vi "Chamber controller Dec 1 2016 no K2420.vi"() -> ()   [LabVIEW 2014]
uses:
  <vilib>/Instr/_visa.llb/VISA Configure Serial Port (Instr).vi
  Environmental Chamber LabVIEW and Instruments/Drivers and Software/Keithley 2100 Series/Public/Configure/Configure 2 Wire Resistance.vi
  <vilib>/Utility/file.llb/Write To Spreadsheet File (string).vi
  <vilib>/Utility/file.llb/Read From Spreadsheet File (string).vi
  Environmental Chamber LabVIEW and Instruments/Drivers and Software/keithley_6430/Keithley 6430/Public/Data/Read (Single Point).vi
  Environmental Chamber LabVIEW and Instruments/Drivers and Software/keithley_6430/Keithley 6430/Keithley 6430.lvlib
  Environmental Chamber LabVIEW and Instruments/Drivers and Software/Keithley 2100 Series/Keithley 2100 Series.lvlib
panel:
  in  "Arduino COMs":T1={"Arduino 1"="COM23", "Arduino 2"="COM24", "Arduino 3"="COM25", "Arduino 4"="COM26", "Arduino 5"="COM27", "Arduino 6"="COM28"}
  out "saving data?":bool
  out "ArduinoQCM\ncluster":T2 caption="Arduino QCM" {"6" format="%_8g"; "5" format="%_8g"; "4" format="%_8g"; "3" format="%_8g"; "2" format="%_8g"; "1" format="%#_10g"}
  in  "Data logging settings":T3={"Save during sequence only"=TRUE, "Save now"=FALSE, "sec between data points"=0.0, "Current data file path"=path "", "Save sample names"={"QCM1"="", "QCM2"="", "QCM3"="", "QCM4"="", "QCM5"="", "QCM6"="", "SRS"="", "K-2420"="", "K-6430"="", "K-2100"=""}, "Experiment Notes"=""} {"sec between data points" min=0.0 max=30.0 format="%#_13g"}
  in  "Sequence cluster":T4={"Save sequence"=FALSE, "Clear sequence"=FALSE, "Import sequence file"=FALSE, "Tare elapsed time"=TRUE, "Run Sequence"=FALSE, "Stop program when sequence ends"=TRUE, "User-defined\nsequence"=[], "Sequence end time"="", "Sequence\npreview"=[], "Current\nstep"=0, "Jump to next step"=FALSE} caption="Sequence settings"
  in  "Pressure parameters cluster":T5={"valve % open"=100.0, "Desired pressure"=0.0, "Vapor sccm"=0.0, "Gas sccm"=0.0, "Valve mode"=enum."% Open", "Pressure Mode"=enum."Abs. pressure", "analyte partial pressure"=23.8, "Turbo pump\nauto on"=TRUE, "Valve position (%)"=0.0, "read pressure"=0.0, "read vapor flow"=0.0, "read gas flow"=0.0, "pressure chart"={"pressure"=0.0}} caption="Pressure settings" {"read gas flow" format="%#_3g"; "read vapor flow" format="%#_3g"; "read pressure" format="%#_7f"; "Valve position (%)" format="%#_3g"; "analyte partial pressure" min=0.0 max=100.0 step=5.0; "Gas sccm" min=0 max=200 step=5; "Vapor sccm" min=0 max=200 step=5; "Desired pressure" min=0.0 max=760.0 step=5.0; "valve % open" min=0.0 max=100.0 step=5.0 format="%#_2f"}
  out "J-KEM temp chart":dbl(graph)
  out "Elapsed time (min)":dbl
  out "State date/time":string caption="Start time"
  out "K-2100 (Ohm)":cluster{"Measurement":dbl}(graph) caption="K-2100"
  out "K-6430":cluster{"Measurement":dbl}(graph)
  out "K-2420":cluster{"Resistance":sgl}(graph)
  in  "Gate time (sec)":enum16{"0.1", "1.0 ", "10"}(ring)=enum."1.0 "
  out "Hz":dbl format="%.7f"
  out "QCM plot":T6(graph)
  in  "Stop":bool
  in  "Clear all charts":bool
  out "O2 sensor output":dbl[](array[numeric]) caption="atm\nTorr"
  in  "rapidox O2 Sensor":bool
  in  "setnag O2 Pump":bool
  in  "Baud Rate 2":i32(ring)=2 items=["2400", "4800", "9600", "19200", "38400", "57600", "115200"]
  in  "Com Port":i32(ring) items=["Com 1", "Com 2", "Com 3", "Com 4", "Com 5", "Com 6", "COM 7", "COM 8", "COM 9", "COM 10", "COM 11", "COM 12", "com 13", "COM 14"]
  in  "Com Port 2":i32(ring) items=["Com 1", "Com 2", "Com 3", "Com 4", "Com 5", "Com 6", "COM 7", "COM 8", "COM 9", "COM 10", "COM 11", "COM 12", "com 13", "COM 14"]
  out "Waveform Chart":cluster{dbl}(graph)
  out "O2 Concentration (PPM)":dbl
  out "Waveform Chart 6":cluster{dbl}(graph)
  # "Currently Unused"
  # "100%"
  # "SRS"
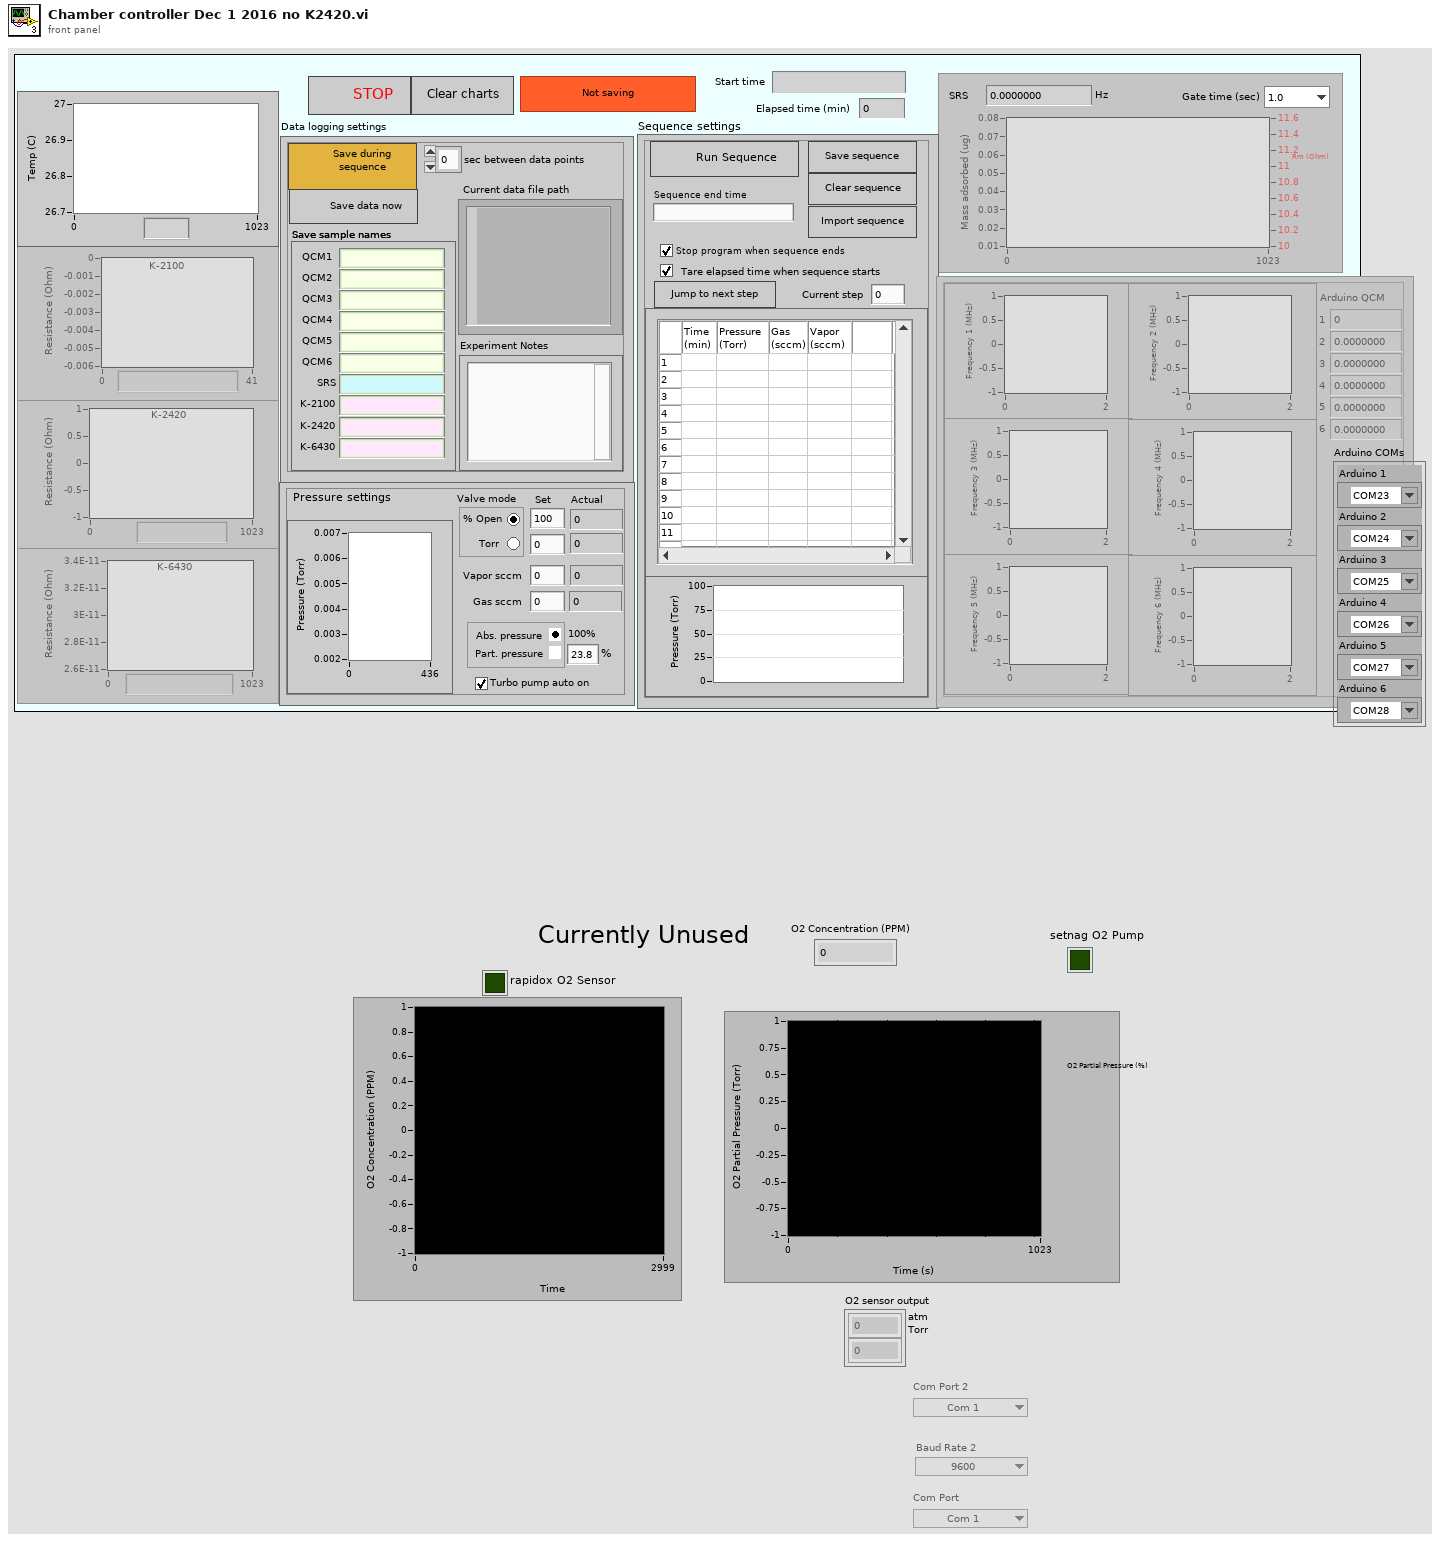
[diagram p1: front panel]
types:
  T1 = cluster{"Arduino 1":refnum<visa-resource-name>, "Arduino 2":refnum<visa-resource-name>, "Arduino 3":refnum<visa-resource-name>, "Arduino 4":refnum<visa-resource-name>, "Arduino 5":refnum<visa-resource-name>, "Arduino 6":refnum<visa-resource-name>}
  T2 = cluster{"arduino qcm 1":dbl, "1":dbl, "arduino qcm 2":dbl, "2":dbl, "arduino qcm 3":dbl, "3":dbl, "arduino qcm 4":dbl, "4":dbl, "arduino qcm 5":dbl, "5":dbl, "arduino qcm 6":dbl, "6":dbl}
  T3 = cluster{"Save during sequence only":bool, "Save now":bool, "sec between data points":dbl, "Current data file path":path, "Save sample names":cluster{"QCM1":string, "QCM2":string, "QCM3":string, "QCM4":string, "QCM5":string, "QCM6":string, "SRS":string, "K-2420":string, "K-6430":string, "K-2100":string}, "Experiment Notes":string}
  T4 = cluster{"Save sequence":bool, "Clear sequence":bool, "Import sequence file":bool, "Tare elapsed time":bool, "Run Sequence":bool, "Stop program when sequence ends":bool, "User-defined\nsequence":string[][], "Sequence end time":string, "Sequence\npreview":cluster{dbl[], dbl[]}[], "Current\nstep":i32, "Jump to next step":bool}
  T5 = cluster{"valve % open":dbl, "Desired pressure":dbl, "Vapor sccm":sgl, "Gas sccm":sgl, "Valve mode":enum32{"% Open", "Torr "}, "Pressure Mode":enum32{"Abs. pressure", " Part. pressure"}, "analyte partial pressure":dbl, "Turbo pump\nauto on":bool, "Valve position (%)":dbl, "read pressure":dbl, "read vapor flow":dbl, "read gas flow":dbl, "pressure chart":cluster{"pressure":dbl}}
  T6 = cluster{"Numeric Control":dbl, "Resistance out":dbl}
  T7 = cluster{"Keithley 6430":bool, "J-KEM":bool, "Keithley 2420":bool, "Keithley 2100":bool, "SRS QCM":bool, "Pressure control":bool, "Arduino":bool}
  T8 = enum8{"Enabled", "Disabled", "Disabled and Grayed Out"}
  T9 = enum16{"open", "open or create", "create or replace", "create", "open (read only)"}
  T10 = enum16{"no parity", "odd parity", "even parity", "mark parity", "space parity"}
  T11 = cluster{"String":string, "String":string, "String":string}
  T12 = cluster{"task out":refnum<k21>, "error out":errorcluster, "task out":refnum<k21>, "error out":errorcluster, "task out":refnum<k21>, "error out":errorcluster, "VISA resource name":refnum<visa-resource-name>, "error out":errorcluster}
  T13 = cluster{"task out":refnum<k21>, "error out":errorcluster, "task out":refnum<k21>, "error out":errorcluster, "task out":refnum<k21>, "error out":errorcluster, "VISA resource name out":refnum<visa-resource-name>, "error out":errorcluster}
  T14 = cluster{bool, "VISA resource name":refnum<visa-resource-name>, "error out":errorcluster}
  T15 = cluster{bool, "VISA resource name out":refnum<visa-resource-name>, "error out":errorcluster}
  T16 = cluster{"VISA resource name out":refnum<visa-resource-name>, "error out":errorcluster, "VISA resource name out":refnum<visa-resource-name>, "error out":errorcluster, "VISA resource name out":refnum<visa-resource-name>, "error out":errorcluster, "VISA resource name out":refnum<visa-resource-name>, "error out":errorcluster, "VISA resource name out":refnum<visa-resource-name>, "error out":errorcluster, "VISA resource name out 2":refnum<visa-resource-name>, "error out 2":errorcluster}
  T17 = cluster{bool, cluster{"task out":refnum<k21>, "error out":errorcluster, "task out":refnum<k21>, "error out":errorcluster, "task out":refnum<k21>, "error out":errorcluster, "VISA resource name out":refnum<visa-resource-name>, "error out":errorcluster}}
  T18 = cluster{"f":dbl, "f":dbl, "f":dbl, "f":dbl, "f":dbl, "f 2":dbl}
  T19 = cluster{"Boolean":bool, "VISA resource name out":refnum<visa-resource-name>, "error out":errorcluster}
  T20 = cluster{bool, "VISA out":refnum<visa-resource-name>, "error out":errorcluster}
  T21 = cluster{"Boolean":bool, "VISA out":refnum<visa-resource-name>, "error out":errorcluster}
  T22 = cluster{"Numeric Control":dbl, "Cluster":cluster{"Numeric Control":dbl}, "String":string, "error out":errorcluster}
  T23 = cluster{bool, "Com Port":i32, "Numeric Control out":dbl}
  T24 = cluster{"Arduino address":refnum<visa-resource-name>, "error in (no error)":errorcluster, "Arduino address 2":refnum<visa-resource-name>, "error in (no error) 2":errorcluster, "Arduino address 3":refnum<visa-resource-name>, "error in (no error) 3":errorcluster, "Arduino address 4":refnum<visa-resource-name>, "error in (no error) 4":errorcluster, "Arduino address 5":refnum<visa-resource-name>, "error in (no error) 5":errorcluster, "Arduino address 6":refnum<visa-resource-name>, "error in (no error) 6":errorcluster}
  T25 = cluster{"mean":string, "mean":string, "mean":string, "mean":string, "mean":string, "mean":string}
  T26 = cluster{"String data out":string, string, string, string}
  T27 = cluster{"valve % open":dbl, "Desired pressure":dbl, "Vapor sccm":sgl, "Gas sccm":sgl, "Valve mode":enum32{"% Open", "Torr "}, "Pressure Mode":enum32{"Abs. pressure", " Part. pressure"}, "analyte partial pressure":dbl, "Turbo pump\nauto on":bool}
  T28 = cluster{"User-defined\nsequence":string[][], "Present (s)":dbl, "current  step # in":i32, "sequence end time in":timestamp}
  T29 = cluster{"current  step # in":i32, "sequence end time in":timestamp, "Boolean":bool}
  T30 = cluster{"press/RH/gas/vapor":cluster{"pressure":string, "RH":string, "gas flow":string, "vapor flow":string}, "Cluster":cluster{"Valve position (%)":dbl, "read pressure":dbl, "read vapor flow":dbl, "read gas flow":dbl}}
  T31 = cluster{"Boolean":bool, "DAQ IDs in":cluster{"task out":refnum<k21>, "error out":errorcluster, "task out":refnum<k21>, "error out":errorcluster, "task out":refnum<k21>, "error out":errorcluster, "VISA Refnum out":refnum<visa-resource-name>, "error out":errorcluster}}
  T32 = cluster{"mean":dbl, "mean":dbl, "mean":dbl, "mean":dbl, "mean":dbl, "mean":dbl}
  T33 = cluster{"f":dbl, "f":dbl, "f":dbl, "f":dbl, "f":dbl}[]
  T34 = cluster{"pressure":string, "RH":string, "gas flow":string, "vapor flow":string}
  T35 = cluster{"Valve position (%)":dbl, "read pressure":dbl, "read vapor flow":dbl, "read gas flow":dbl}
  T36 = cluster{"mean":dbl, "mean":dbl, "mean":dbl, "mean":dbl, "mean":dbl, "mean":dbl, "mean":dbl, "mean":dbl, "mean":dbl, "mean":dbl, "mean":dbl, "mean":dbl}
  T37 = cluster{"QCM1":string, "QCM2":string, "QCM3":string, "QCM4":string, "QCM5":string, "QCM6":string, "SRS":string, "K-2420":string, "K-6430":string, "K-2100":string}
  T38 = cluster{"task out":refnum<k21>, "error out":errorcluster, "task out":refnum<k21>, "error out":errorcluster, "task out":refnum<k21>, "error out":errorcluster, "VISA Refnum out":refnum<visa-resource-name>, "error out":errorcluster}
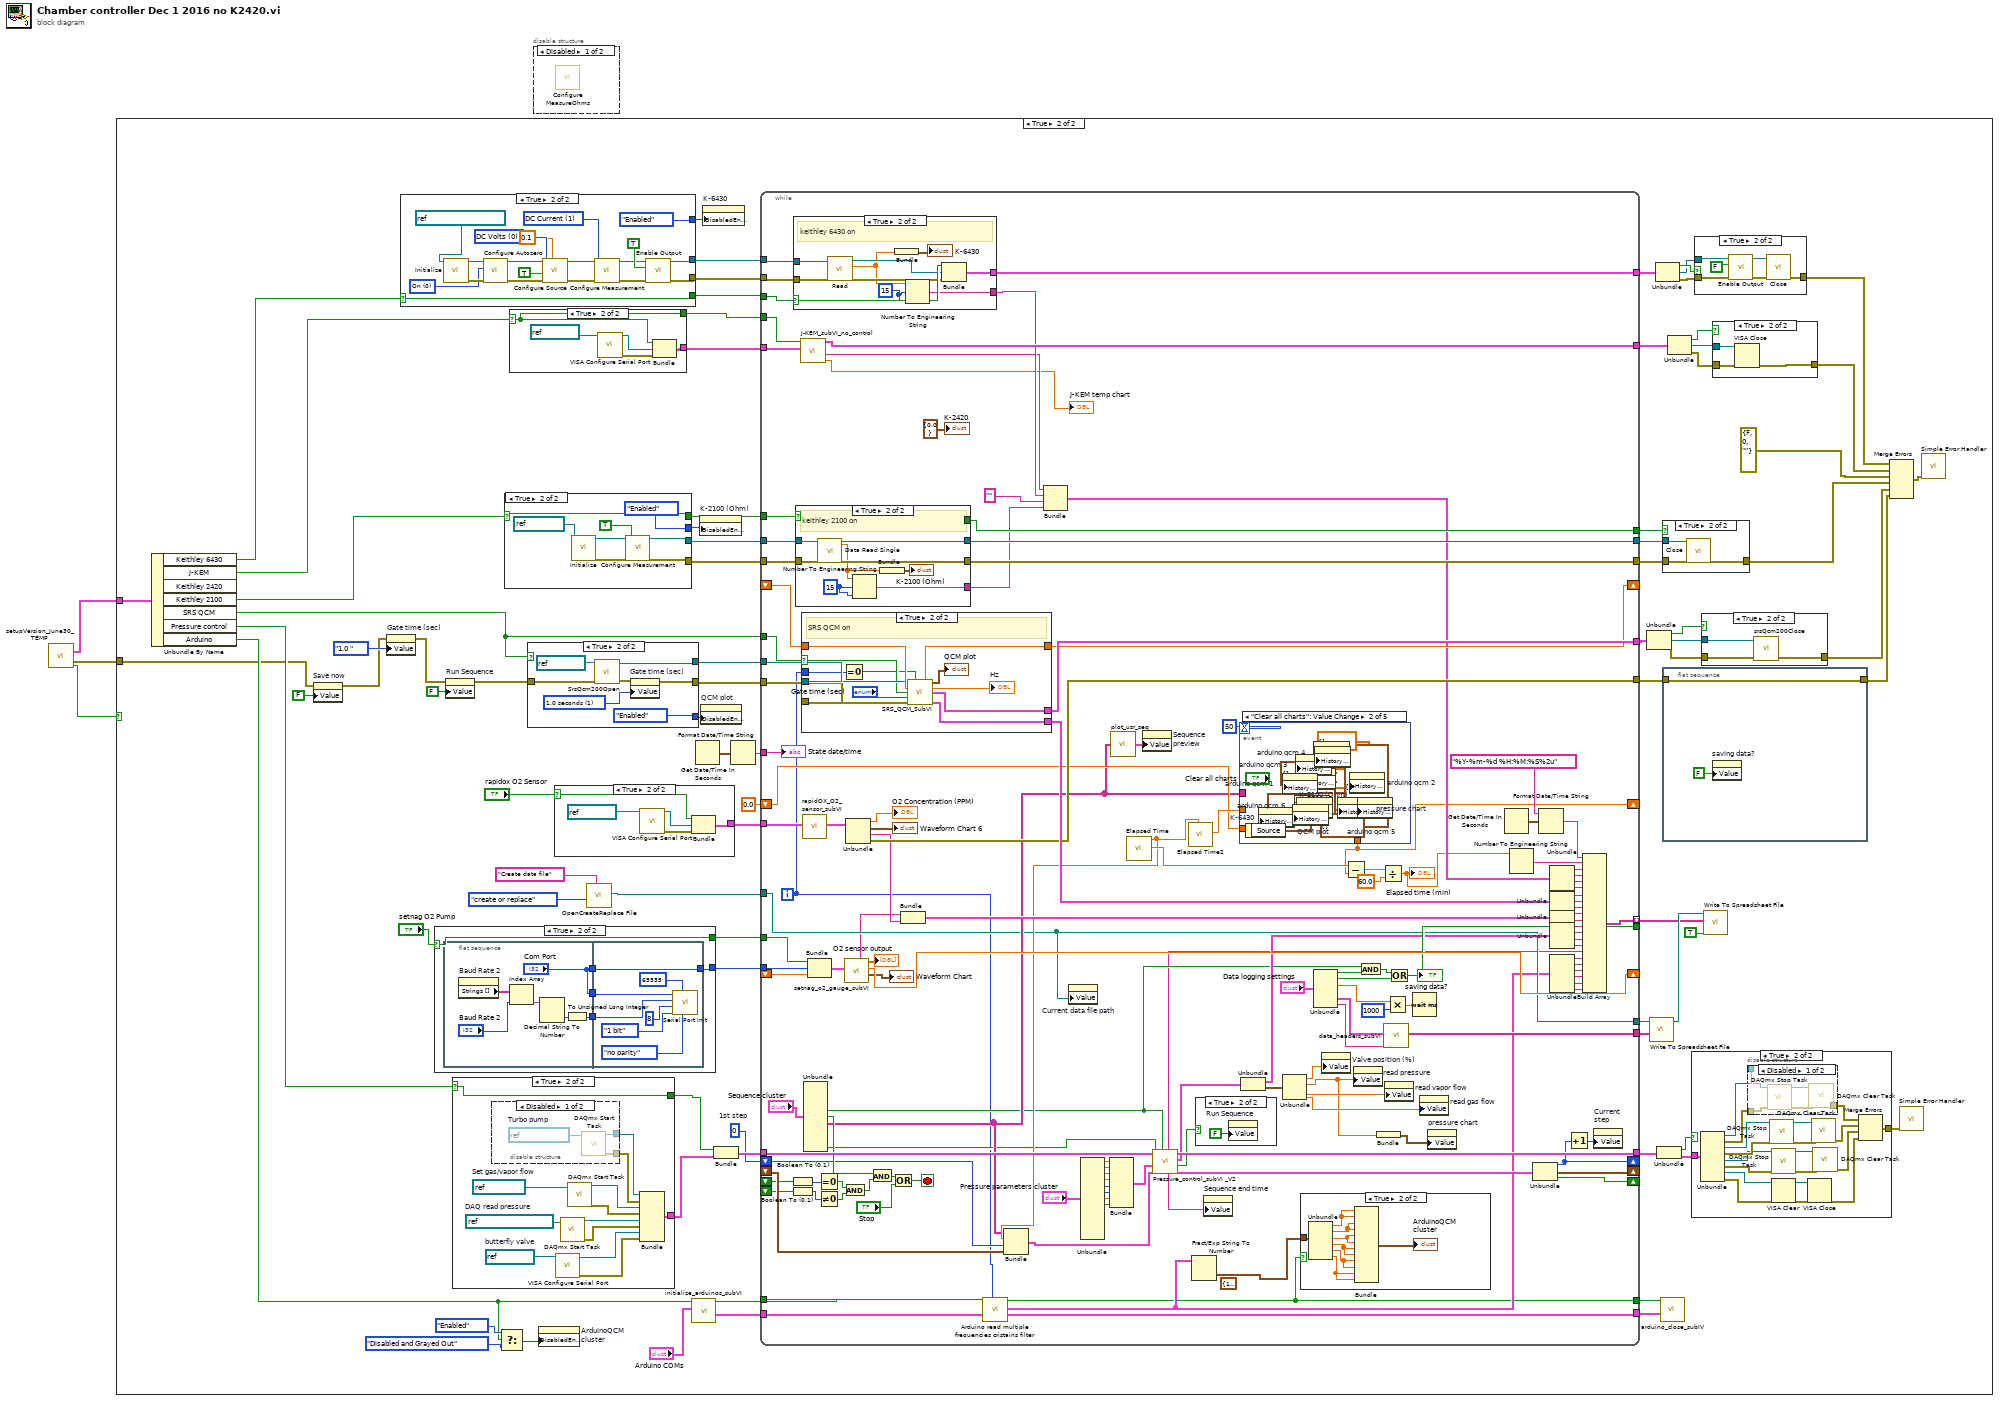
[diagram p0: block diagram]
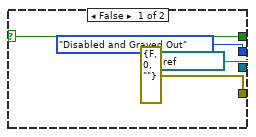
[diagram p5: hidden frame]
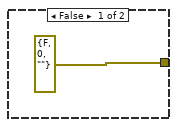
[diagram p6: hidden frame]
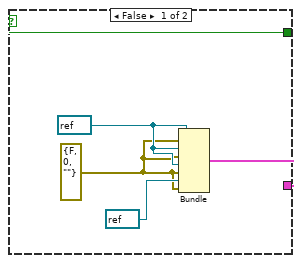
[diagram p8: hidden frame]
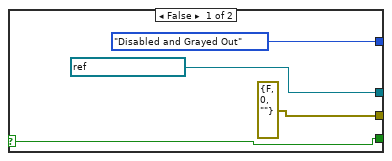
[diagram p11: hidden frame]
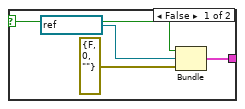
[diagram p12: hidden frame]
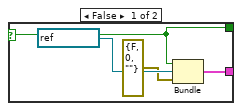
[diagram p14: hidden frame]
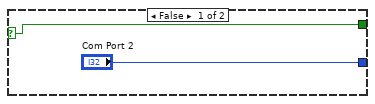
[diagram p15: hidden frame]
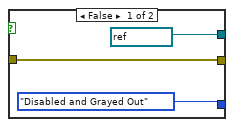
[diagram p17: hidden frame]
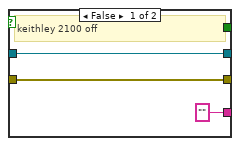
[diagram p20: hidden frame]
diagram:
  n1 = call "setupVersion_June30_TEMP.vi"() -> ("Instruments on/off"=w1:T7, "error IO"=w2:errorcluster, "OK"=w3:bool)  [unwired: 13 in]
  n2 = case shown="True" w3 {
    tunnel: w2 -> [_ w9]
    tunnel: w1 -> [_ w16]
    frame False {
    }
    frame True {
      w28 = 0  # 1st step
      n3 = Unbundle By Name(w16) -> ("Keithley 6430"=w15:bool, "J-KEM"=w14:bool, "Keithley 2100"=w13:bool, "SRS QCM"=w12:bool, "Pressure control"=w11:bool, "Arduino"=w10:bool)  [unwired: 1 out]
      n4 = property on="Save now" class="Bool (strict)"(error in=w9, "Value"=FALSE) -> (error out=w8:errorcluster)  [unwired: 1 in, 1 out]
      n5 = property on="Gate time (sec)" class="Enum (strict)"(error in=w8, "Value"=enum16{"0.1", "1.0 ", "10"}."1.0 " ("Gate time (sec)")) -> (error out=w17:errorcluster)  [unwired: 1 in, 1 out]
      n6 = case shown="True" w15 {
        selector: w15 -> [w158 w168]
        tunnel: [refnum<visa-resource-name> "GPIB0::29::INSTR" ("VISA resource name") w177] -> w59
        tunnel: [errorcluster {"status"=FALSE, "code"=0, "source"=""} ("error out") w178] -> w58
        tunnel: [T8."Disabled and Grayed Out" ("Disabled") T8."Enabled" ("Disabled")] -> w53
        tunnel: [w158 w168] -> w47
        frame False {
        }
        frame True {
          w163 = u16 1 items=["DC Volts", "DC Current"] ("Measure Function (1: DC Current)")
          w169 = u16 0 items=["DC Volts", "DC Current"] ("Source Function (0: DC Volts)")
          w174 = u16 0 items=["On", "Off", "Once"] ("Autozero  (0: On)")
          n7 = call "Initialize.vi"("VISA resource name"=refnum<visa-resource-name> "GPIB0::29::INSTR") -> ("error out"=w175:errorcluster, "VISA resource name out"=w176:refnum<visa-resource-name>)  [unwired: 4 in, 5 out]
          n8 = call "Configure Autozero.vi"("error in (no error)"=w175, "Autozero  (0: On)"=w174, "VISA resource name"=w176) -> ("error out"=w171:errorcluster, "VISA resource name out"=w172:refnum<visa-resource-name>)  [unwired: 7 in]
          n9 = call "Configure Source.vi"("V-Source Level [V]"=0.1, "error in (no error)"=w171, "Auto Range (T:Enable)"=TRUE, "Source Function (0: DC Volts)"=w169, "VISA resource name"=w172) -> ("error out"=w165:errorcluster, "VISA resource name out"=w167:refnum<visa-resource-name>)  [unwired: 5 in]
          n10 = call "Configure Measurement.vi"("error in (no error)"=w165, "Measure Function (1: DC Current)"=w163, "VISA resource name"=w167) -> ("error out"=w164:errorcluster, "VISA resource name out"=w166:refnum<visa-resource-name>)  [unwired: 7 in]
          n11 = call "Enable Output.vi"("error in (no error)"=w164, "Enable Output (F:Off)"=TRUE ("Output (F:Off)"), "VISA resource name"=w166) -> ("error out"=w178:errorcluster, "VISA resource name out"=w177:refnum<visa-resource-name>)  [unwired: 7 out]
        }
      }
      n12 = case shown="True" "setnag O2 Pump" {
        selector: "setnag O2 Pump" -> [w203 w205]
        tunnel: ["Com Port 2" w206] -> w81
        tunnel: [w203 w205] -> w36
        frame False {
        }
        frame True {
          n13 = flat-sequence {
            tunnel: ["Com Port"] -> w209
            tunnel: [w211] -> w208
            tunnel: ["Com Port"] -> w207
            tunnel: w209 -> [w217]
            tunnel: w208 -> [w216]
            tunnel: w207 -> [w218]
            tunnel: [w218] -> w206
            frame #0 {
              n14 = property on="Baud Rate 2" class="Ring (strict)"() -> ("Strings []"=w213:string[])  [unwired: 2 in, 2 out]
              n15 = Index Array(array=w213, index="Baud Rate 2") -> (element=w214:string)
              n16 = Decimal String To Number(string=w214) -> (number=w212:i32)  [unwired: 2 in, 1 out]
              n17 = To Unsigned Long Integer(number=w212) -> (unsigned 32bit integer=w211:u32)
            }
            frame #1 {
              n18 = call <vilib>:"Serial Port Init.vi"("parity"=T10."no parity", "buffer size"=u16 65535, "stop bits"=enum16{"1 bit", "1.5 bits", "2 bits"}."1 bit", "data bits"=u16 8, "baud rate"=w216, "port number"=w217) -> ()  [unwired: 1 in, 1 out]
            }
          }
        }
      }
      n19 = property on="Run Sequence" class="Bool (strict)"(error in=w17, "Value"=FALSE) -> (error out=w23:errorcluster)  [unwired: 1 in, 1 out]
      n20 = case shown="True" w11 {
        selector: w11 -> [w130 w135]
        tunnel: [w131 w137] -> w30
        tunnel: [w130 w135] -> w31
        frame False {
          w133 = refnum<k21> refnum ("task out")
          w132 = errorcluster {"status"=FALSE, "code"=0, "source"=""} ("error out")
          n21 = Bundle("task out"=w133, "error out"=w132, "task out"=w133, "error out"=w132, "task out"=w133, "error out"=w132, "VISA resource name"=refnum<visa-resource-name> refnum, "error out"=w132) -> (w131:T12)  [unwired: 1 in]
        }
        frame True {
          w145 = refnum<visa-resource-name> "COM5"  # butterfly valve
          w146 = refnum<k21> "Setflow"  # Set gas/vapor flow
          w147 = refnum<k21> "AllDaqReadings"  # DAQ read pressure
          n22 = disable-structure shown="Disabled" {
            disable-tunnel: [w149 _] -> w144
            disable-tunnel: [w148 _] -> w143
            frame Disabled {
              w150 = refnum<k21> "TurboON"  # Turbo pump
              n23 = call <vilib>:"DAQmx Start Task.vi"("task/channels in"=w150) -> ("task out"=w149:refnum<k21>, "error out"=w148:errorcluster)  [unwired: 13 in]
            }
            frame Enabled {
            }
          }
          n24 = call-poly "VISA Configure Serial Port"("VISA resource name"=w145) -> ("VISA resource name out"=w138:refnum<visa-resource-name>, "error out"=w136:errorcluster)  [unwired: 13 in]
          n25 = call <vilib>:"DAQmx Start Task.vi"("task/channels in"=w147) -> ("task out"=w140:refnum<k21>, "error out"=w139:errorcluster)  [unwired: 13 in]
          n26 = call <vilib>:"DAQmx Start Task.vi"("task/channels in"=w146) -> ("task out"=w142:refnum<k21>, "error out"=w141:errorcluster)  [unwired: 13 in]
          n27 = Bundle("task out"=w144, "error out"=w143, "task out"=w142, "error out"=w141, "task out"=w140, "error out"=w139, "VISA resource name out"=w138, "error out"=w136) -> (w137:T13)  [unwired: 1 in]
        }
      }
      n28 = Select(t=T8."Enabled" ("Disabled"), s=w10, f=T8."Disabled and Grayed Out" ("Disabled")) -> (s? t:f=w22:T8)
      n29 = case shown="True" w13 {
        selector: w13 -> [w93 w98]
        tunnel: [refnum<visa-resource-name> "K-2100" ("VISA resource name out") w101] -> w45
        tunnel: [errorcluster {"status"=FALSE, "code"=0, "source"=""} ("error out") w100] -> w44
        tunnel: [w93 w98] -> w43
        tunnel: [T8."Disabled and Grayed Out" ("Disabled") T8."Enabled" ("Disabled")] -> w38
        frame False {
        }
        frame True {
          n30 = call "Initialize.vi"("VISA resource name"=refnum<visa-resource-name> "K-2100") -> ("VISA resource name out"=w102:refnum<visa-resource-name>, "error out"=w99:errorcluster)  [unwired: 17 in]
          n31 = call-poly "Configure Measurement.vi"("VISA resource name"=w102, "error in (no error)"=w99, "Auto Range? (T: Auto)"=TRUE) -> ("VISA resource name out"=w101:refnum<visa-resource-name>, "error out"=w100:errorcluster)  [unwired: 15 in]
        }
      }
      n32 = case shown="True" w14 {
        selector: w14 -> [w194 w199]
        tunnel: [w195 w200] -> w75
        tunnel: [w194 w199] -> w69
        frame False {
          n33 = Bundle(w194, "VISA resource name"=refnum<visa-resource-name> "COM3", "error out"=errorcluster {"status"=FALSE, "code"=0, "source"=""}) -> (w195:T14)  [unwired: 1 in]
        }
        frame True {
          n34 = call-poly "VISA Configure Serial Port"("VISA resource name"=refnum<visa-resource-name> "COM3") -> ("VISA resource name out"=w201:refnum<visa-resource-name>, "error out"=w198:errorcluster)  [unwired: 13 in]
          n35 = Bundle(w199, "VISA resource name out"=w201, "error out"=w198) -> (w200:T15)  [unwired: 1 in]
        }
      }
      n36 = case shown="True" w12 {
        tunnel: [refnum<visa-resource-name> "COM6" ("VISA in") w233] -> w83
        tunnel: [w228 w230] -> w82
        tunnel: w23 -> [w228 w235]
        tunnel: [T8."Disabled and Grayed Out" ("Disabled") T8."Enabled" ("Disabled")] -> w54
        frame False {
        }
        frame True {
          w232 = u16 1 items=["0.1 seconds", "1.0 seconds", "10.0 seconds"] ("Gate time")
          n37 = call "SrsQcm200Open.vi"("error in"=w235, "VISA in"=refnum<visa-resource-name> "COM6") -> ("error out"=w231:errorcluster, "VISA out"=w233:refnum<visa-resource-name>)  [unwired: 3 in]
          n38 = property on="Gate time (sec)" class="Enum (strict)"(error in=w231, "Value"=w232) -> (error out=w230:errorcluster)  [unwired: 1 in, 1 out]
        }
      }
      n39 = property on="ArduinoQCM\ncluster" class="Clust (strict)"("DisabledEnum"=w22) -> ()  [unwired: 2 in, 2 out]
      n40 = case shown="True" "rapidox O2 Sensor" {
        selector: "rapidox O2 Sensor" -> [w181 w186]
        tunnel: [w182 w187] -> w65
        frame False {
          n41 = Bundle(w181, "VISA resource name"=refnum<visa-resource-name> "COM7", "error out"=errorcluster {"status"=FALSE, "code"=0, "source"=""}) -> (w182:T14)  [unwired: 1 in]
        }
        frame True {
          n42 = call-poly "VISA Configure Serial Port"("VISA resource name"=refnum<visa-resource-name> "COM7") -> ("VISA resource name out"=w188:refnum<visa-resource-name>, "error out"=w185:errorcluster)  [unwired: 13 in]
          n43 = Bundle(w186, "VISA resource name out"=w188, "error out"=w185) -> (w187:T15)  [unwired: 1 in]
        }
      }
      n44 = call "OpenCreateReplace File.vi"("prompt"="Create data file", "function (open:0)"=T9."create or replace") -> ("new file path"=w46:path)  [unwired: 6 in, 3 out]
      n45 = call "initialize_arduinos_subVI.vi"("arduino 1-6 addresses"="Arduino COMs", "arduinos on?"=w10) -> ("arduino addresses/errors"=w32:T16, "arduinos on/off"=w51:bool)  [unwired: 8 in]
      n46 = Get Date/Time In Seconds() -> (seconds since 1Jan1904=w85:timestamp)
      n47 = property on="K-2100 (Ohm)" class="WFChart (strict)"("DisabledEnum"=w38) -> ()  [unwired: 2 in, 2 out]
      n48 = property on="QCM plot" class="WFChart (strict)"("DisabledEnum"=w54) -> ()  [unwired: 2 in, 2 out]
      n49 = property on="K-6430" class="WFChart (strict)"("DisabledEnum"=w53) -> ()  [unwired: 2 in, 2 out]
      n50 = Bundle(w31, w30) -> (w29:T17)  [unwired: 1 in]
      n51 = Format Date/Time String(seconds (now)=w85) -> (date/time string=w35:string)  [unwired: 2 in]
      n52 = while {
        shift-right: [w377] -> _
        shift-left: _ -> [w313]
        tunnel: [w365] -> w52 mode=indexing if=w334
        tunnel: w83 -> [w376]
        tunnel: w82 -> [w375]
        tunnel: w12 -> [w374]
        tunnel: w36 -> [w315]
        tunnel: w81 -> [w316]
        tunnel: [w373] -> w79
        tunnel: w75 -> [w372]
        tunnel: [w371] -> w74
        tunnel: w69 -> [w370]
        tunnel: w65 -> [w323]
        tunnel: [w319] -> w6
        tunnel: [w255] -> w64
        tunnel: w46 -> [w255]
        shift-right: [w363] -> _
        shift-left: _ -> [w364]
        tunnel: w59 -> [w369]
        tunnel: w58 -> [w368]
        tunnel: [w367] -> w57
        tunnel: [w334] -> _
        tunnel: w51 -> [w242]
        tunnel: w32 -> [w245]
        tunnel: [w241] -> w49
        tunnel: [w243] -> w50
        tunnel: [w351] -> w48
        tunnel: w47 -> [w346]
        tunnel: w45 -> [w333]
        tunnel: w44 -> [w332]
        tunnel: w43 -> [w331]
        tunnel: [w330] -> w42
        tunnel: [w329] -> w41
        tunnel: [w328] -> w40
        shift-right: [w307] -> _
        shift-left: 0.0 ("Elapsed Time (s)") -> [w308]
        tunnel: w35 -> [w298]
        tunnel: w29 -> [w280]
        shift-right: [w250] -> _
        shift-left: w28 -> [w269]
        shift-right: [w275] -> _
        shift-left: _ -> [w273]
        shift-right: [w274] -> _
        shift-left: _ -> [w272]
        shift-left: _ -> [w271]
        tunnel: [w267] -> w27
        i -> [w240]
        stop <- w336 stop-if-true
        (unwired) T18 {"f"=1000000.0, "f"=1000000.0, "f"=1000000.0, "f"=1000000.0, "f"=1000000.0, "f 2"=1000000.0} ("y")
        n53 = Boolean To (0,1)(Boolean=w272) -> (0, 1=w344:i16)
        n54 = Boolean To (0,1)(Boolean=w271) -> (0, 1=w343:i16)
        n55 = case "Keithley 6430" shown="True" w346 {
          selector: w346 -> [w412 w423]
          tunnel: w369 -> [w411 w420]
          tunnel: w368 -> [w410 w419]
          tunnel: ["" w422] -> w318
          tunnel: [w409 w421] -> w367
          frame False {
            # "keithley 6430 off"
            n56 = Bundle(w412, "VISA resource name out"=w411, "error out"=w410) -> (w409:T15)  [unwired: 1 in]
          }
          frame True {
            w414 = i16 15 ("width (-)")
            # "keithley 6430 on"
            n57 = call-poly "Read.vi"("error in (no error)"=w419, "VISA resource name"=w420) -> ("error out"=w418:errorcluster, "Measurement"=w416:dbl, "VISA resource name out"=w417:refnum<visa-resource-name>)  [unwired: 1 in, 6 out]
            n58 = Bundle("Measurement"=w416) -> (→"K-6430":cluster{"Measurement":dbl})  [unwired: 1 in]
            n59 = Number To Engineering String(2:w414, 3:w414, 4:w416) -> (0:w422:string)  [unwired: 1 in]
            n60 = Bundle(w423, "VISA resource name out"=w417, "error out"=w418) -> (w421:T15)  [unwired: 1 in]
          }
        }
        n61 = case shown="True" w331 {
          selector: w331 -> [w388 w393]
          tunnel: [w389 w400] -> w329
          tunnel: [w390 w399] -> w328
          tunnel: w333 -> [w389 w398]
          tunnel: w332 -> [w390 w397]
          tunnel: ["" w395] -> w317
          tunnel: [w388 w393] -> w330
          frame False {
            # "keithley 2100 off"
          }
          frame True {
            w392 = i16 15 ("width (-)")
            # "keithley 2100 on"
            n62 = call "Data Read Single.vi"("VISA resource name"=w398, "error in (no error)"=w397) -> ("VISA resource name out"=w400:refnum<visa-resource-name>, "Measurement"=w396:dbl, "error out"=w399:errorcluster)  [unwired: 15 in]
            n63 = Number To Engineering String ("elapsed time (min)")(2:w392, 3:w392, 4:w396) -> (0:w395:string)  [unwired: 1 in]
            n64 = Bundle("Measurement"=w396) -> (→"K-2100 (Ohm)":cluster{"Measurement":dbl})  [unwired: 1 in]
          }
        }
        n65 = call "J-KEM_subVI_no_control.vi"("Address in"=w372, "J-KEM on?"=w370) -> ("Temp (C)"=→"J-KEM temp chart":dbl, "String data out"=w306:string, "Address out"=w371:T19)  [unwired: 6 in, 1 out]
        n66 = case "SRS QCM" shown="True" w374 {
          selector: w374 -> [w426 w435]
          tunnel: w376 -> [w429 w437]
          tunnel: w375 -> [w428 w438]
          tunnel: [w427 w441] -> w373
          tunnel: w364 -> [w424 w440]
          tunnel: [w424 w439] -> w363
          tunnel: [T11 {"String"="", "String"="", "String"=""} ("M,F,MR output cluster") w434] -> w356
          tunnel: w240 -> [_ w431]
          frame False {
            # "SRS QCM off"
            n67 = Bundle(w426, "VISA out"=w429, "error out"=w428) -> (w427:T20)  [unwired: 1 in]
          }
          frame True {
            # "SRS QCM on"
            n68 = Equal To 0?(x=w431) -> (x = 0?=w432:bool)
            n69 = call "SRS_QCM_SubVI.vi"("VISA Refnum in"=w437, "first iteration?"=w432, "Frequency out 3"=w440, "Boolean 2"=w435, "Gate time"="Gate time (sec)", "error in (no error)"=w438) -> ("Frequency out 2"=w439:dbl, "Cluster"=→"QCM plot":T6, "Frequency out"=→"Hz":dbl, "Cluster 2"=w441:T21, "M,F,MR output cluster"=w434:T11)  [unwired: 2 in, 3 out]
          }
        }
        n70 = call "rapidOX_O2_sensor_subVI.vi"("rapid ox info in"=w323) -> ("rapidox info out"=w322:T22)  [unwired: 10 in]
        n71 = Unbundle("Sequence cluster") -> ("Run Sequence"=w261:bool, "Stop program when sequence ends"=w270:bool, "User-defined\nsequence"=w265:string[][], "Jump to next step"=w251:bool)  [unwired: 7 out]
        n72 = Bundle(w315, "Com Port"=w316, "Numeric Control out"=w313) -> (w314:T23)  [unwired: 1 in]
        n73 = Equal To 0?(x=w344) -> (x = 0?=w341:bool)
        n74 = Not Equal To 0?(x=w343) -> (x != 0?=w342:bool)
        n75 = And(x=w341, y=w342) -> (x .and. y?=w335:bool)
        n76 = call "setnag_o2_gauge_subVI.vi"("setnag info in"=w314) -> ("Cluster"=→"Waveform Chart":cluster{"Numeric Control":dbl}, "Numeric Control out"=w377:dbl, "Array"=→"O2 sensor output":dbl[], "String"=w252:string)  [unwired: 7 in]
        n77 = Unbundle(w322) -> ("Numeric Control"=→"O2 Concentration (PPM)":dbl, "Cluster"=→"Waveform Chart 6":cluster{"Numeric Control":dbl}, "String"=w297:string, "error out"=w319:errorcluster)
        n78 = And(x=w270, y=w335) -> (x .and. y?=w311:bool)
        n79 = Or(x=w311, y="Stop") -> (x .or. y?=w336:bool)
        n80 = Bundle("String"=w252, "String"=w297) -> (w296:cluster{"String":string, "String":string})  [unwired: 1 in]
        n81 = call "Arduino read multiple frequencies cristains filter.vi"("main loop iteration number"=w240, "arduino addresses in"=w245, "arduinos on?"=w242) -> ("arduino addresses out"=w243:T24, "arduino frequencies out"=w244:T25, "arduinos on"=w241:bool)  [unwired: 6 in]
        n82 = Bundle("String data out"=w306, w318, "", w317) -> (w312:T26)  [unwired: 1 in]
        n83 = property on="Current data file path" class="Path"("Value"=w255) -> ()  [unwired: 2 in, 2 out]
        n84 = Unbundle("Pressure parameters cluster") -> ("valve % open"=w285:dbl, "Desired pressure"=w287:dbl, "Vapor sccm"=w288:sgl, "Gas sccm"=w289:sgl, "Valve mode"=w290:enum32{"% Open", "Torr "}, "Pressure Mode"=w291:enum32{"Abs. pressure", " Part. pressure"}, "analyte partial pressure"=w292:dbl, "Turbo pump\nauto on"=w293:bool)  [unwired: 5 out]
        n85 = Bundle("valve % open"=w285, "Desired pressure"=w287, "Vapor sccm"=w288, "Gas sccm"=w289, "Valve mode"=w290, "Pressure Mode"=w291, "analyte partial pressure"=w292, "Turbo pump\nauto on"=w293) -> (w284:T27)  [unwired: 1 in]
        n86 = call "plot_usr_seq.vi"("User-defined sequence"=w265) -> ("Sequence Preview"=w257:cluster{dbl[], dbl[]}[])
        n87 = call "Elapsed Time"() -> ("Present (s)"=w277:dbl, "Elapsed Time (s)"=w325:dbl)  [unwired: 12 in, 6 out]
        n88 = Bundle("User-defined\nsequence"=w265, "Present (s)"=w277, "current  step # in"=w269, "sequence end time in"=w273) -> (w278:T28)  [unwired: 1 in]
        n89 = property on="Sequence\npreview" class="XYGraph (strict)"("Value"=w257) -> ()  [unwired: 2 in, 2 out]
        n90 = call "Pressure_control_subVI _V2.vi"("Run Sequence"=w261, "user sequence, present (s) in, current step in, seq time in"=w278, "pressure parameters in"=w284, "Jump to next step"=w251, "pressure control on? / DAQ IDs/errors in"=w280) -> ("current step # out, shift register time out, seq button on?"=w276:T29, "sequence over? USE THIS TO REINITIALIZE RUN SEQUENCE BUTTON SO PROGRAM ENDS"=w266:bool, "save press/RH/gasflow/vaporflow - read valve position/pressure/vaporflow/gasflow"=w264:T30, "pressure control on out, DAQ IDs/errors out"=w267:T31, "sequence end date/time string"=w268:string, "pressure_setpoint"=w247:string)  [unwired: 1 in]
        n91 = call "Elapsed Time2"("Set Start Time (s)"=w277) -> ("Elapsed Time (s)"=w309:dbl)  [unwired: 11 in, 7 out]
        n92 = Fract/Exp String To Number(string=w244) -> (number=w239:T32)  [unwired: 3 in, 1 out]
        n93 = case shown="True" w266 {
          frame False {
          }
          frame True {
            n94 = property on="Run Sequence" class="Bool (strict)"("Value"=FALSE ("Run Sequence")) -> ()  [unwired: 2 in, 2 out]
          }
        }
        n95 = property on="Sequence end time" class="Str"("Value"=w268) -> ()  [unwired: 2 in, 2 out]
        n96 = event shown="[1] \"Clear all charts\": Value Change" {
          selector: _ -> [_ _ _ _ _]
          dyn-events: _ -> [_ _ _ _ _]
          timeout: 50 -> [_ _ _ _ _]
          tunnel: w265 -> [_ _ _ w407 _]
          tunnel: w309 -> [_ _ _ _ _]
          tunnel: w308 -> [w401 _ _ _ _]
          tunnel: [w401 _ _ _ _] -> w307
          event Timeout {
            n97 = event-data() -> ()  [unwired: 1 in, 1 out]
          }
          event "Clear all charts": Value Change {
            (unwired) T33 [] ("History Data")
            w404 = cluster{dbl}[] [] ("History Data")
            w405 = cluster{"Resistance":sgl}[] [] ("History Data")
            w402 = dbl[] [] ("History Data")
            n98 = event-data() -> ()  [unwired: 1 in, 1 out]
            n99 = property on="K-6430" class="WFChart (strict)"("History Data"=w405) -> ()  [unwired: 2 in, 2 out]
            n100 = property on="arduino qcm 1" class="WFChart (strict)"("History Data"=w402) -> ()  [unwired: 2 in, 2 out]
            n101 = property on="Waveform Chart" class="WFChart (strict)"("History Data"=w404) -> ()  [unwired: 2 in, 2 out]
            n102 = property on="arduino qcm 6" class="WFChart (strict)"("History Data"=w402) -> ()  [unwired: 2 in, 2 out]
            n103 = property on="arduino qcm 3" class="WFChart (strict)"("History Data"=w402) -> ()  [unwired: 2 in, 2 out]
            n104 = property on="QCM plot" class="WFChart (strict)"("History Data"=cluster{dbl, "Resistance out":dbl}[] []) -> ()  [unwired: 2 in, 2 out]
            n105 = property on="K-2100 (Ohm)" class="WFChart (strict)"("History Data"=w405) -> ()  [unwired: 2 in, 2 out]
            n106 = property on="arduino qcm 4" class="WFChart (strict)"("History Data"=w402) -> ()  [unwired: 2 in, 2 out]
            n107 = property on="K-2420" class="WFChart (strict)"("History Data"=w405) -> ()  [unwired: 2 in, 2 out]
            n108 = property on="pressure chart" class="WFChart (strict)"("History Data"=w404) -> ()  [unwired: 2 in, 2 out]
            n109 = property on="arduino qcm 2" class="WFChart (strict)"("History Data"=w402) -> ()  [unwired: 2 in, 2 out]
            n110 = property on="arduino qcm 5" class="WFChart (strict)"("History Data"=w402) -> ()  [unwired: 2 in, 2 out]
          }
          event "Sequence cluster.Clear sequence": Value Change {
            n111 = event-data() -> ()  [unwired: 1 in, 1 out]
            n112 = property on="User-defined\nsequence" class="Tbl (strict)"("Value"=string[][] []) -> ()  [unwired: 2 in, 2 out]
          }
          event "Sequence cluster.Save sequence": Value Change {
            n113 = event-data() -> ()  [unwired: 1 in, 1 out]
            n114 = call-poly <vilib>:"Write To Spreadsheet File.vi"("2D data"=w407) -> ()  [unwired: 7 in, 1 out]
          }
          event "Sequence cluster.Import sequence file": Value Change {
            n115 = event-data() -> ()  [unwired: 1 in, 1 out]
            n116 = call-poly <vilib>:"Read From Spreadsheet File.vi"() -> ("all rows"=w408:string[][])  [unwired: 7 in, 4 out]
            n117 = property on="User-defined\nsequence" class="Tbl (strict)"("Value"=w408) -> ()  [unwired: 2 in, 2 out]
          }
        }
        n118 = Unbundle(w264) -> ("press/RH/gas/vapor"=w263:T34, "Cluster"=w262:T35)
        n119 = Unbundle(w262) -> ("Valve position (%)"=w260:dbl, "read pressure"=w254:dbl, "read vapor flow"=w259:dbl, "read gas flow"=w258:dbl)
        n120 = case shown="True" w241 {
          tunnel: w239 -> [_ w387]
          frame False {
          }
          frame True {
            n121 = Unbundle(w387) -> ("mean"=w386:dbl, "mean"=w385:dbl, "mean"=w384:dbl, "mean"=w383:dbl, "mean"=w382:dbl, "mean"=w380:dbl)
            n122 = Bundle("mean"=w386, "mean"=w386, "mean"=w385, "mean"=w385, "mean"=w384, "mean"=w384, "mean"=w383, "mean"=w383, "mean"=w382, "mean"=w382, "mean"=w380, "mean"=w380) -> (→"ArduinoQCM\ncluster":T36)  [unwired: 1 in]
          }
        }
        n123 = Unbundle("Data logging settings") -> ("Save during sequence only"=w338:bool, "Save now"=w340:bool, "sec between data points"=w327:dbl, "Save sample names"=w282:T37, "Experiment Notes"=w281:string)  [unwired: 1 out]
        n124 = property on="Valve position (%)" class="DigNum (strict)"("Value"=w260) -> ()  [unwired: 2 in, 2 out]
        n125 = Subtract(x=w325, y=w307) -> (x-y=w324:dbl)
        n126 = property on="read pressure" class="DigNum (strict)"("Value"=w254) -> ()  [unwired: 2 in, 2 out]
        n127 = And(x=w261, y=w338) -> (x .and. y?=w337:bool)
        n128 = Bundle("read pressure"=w254) -> (w253:cluster{"read pressure":dbl})  [unwired: 1 in]
        n129 = Divide(x=w324, y=60.0) -> (x/y=w299:dbl)
        "Elapsed time (min)" <- w299
        n130 = call "data_headers_subVI.vi"("Experiment Notes"=w281, "Sample names"=w282) -> ("data headers"=w351:string[])  [unwired: 9 in]
        n131 = property on="read vapor flow" class="DigNum (strict)"("Value"=w259) -> ()  [unwired: 2 in, 2 out]
        n132 = Multiply(x=w327, y=u32 1000 ("x")) -> (x*y=w360:dbl)
        n133 = Or(x=w337, y=w340) -> (x .or. y?=w334:bool)
        "saving data?" <- w334
        n134 = Wait (ms)(milliseconds to wait=w360) -> ()  [unwired: 1 out]
        n135 = property on="read gas flow" class="DigNum (strict)"("Value"=w258) -> ()  [unwired: 2 in, 2 out]
        n136 = property on="pressure chart" class="WFChart (strict)"("Value"=w253) -> ()  [unwired: 2 in, 2 out]
        n137 = Get Date/Time In Seconds() -> (seconds since 1Jan1904=w378:timestamp)
        n138 = Number To Engineering String ("elapsed time (min)")(4:w299) -> (0:w304:string)  [unwired: 3 in]
        n139 = Unbundle(w276) -> ("current  step # in"=w250:i32, "sequence end time in"=w275:timestamp, "Boolean"=w274:bool)
        n140 = Format Date/Time String(time format string (%c)="%Y-%m-%d %H:%M:%S%2u", seconds (now)=w378) -> (date/time string=w357:string)  [unwired: 1 in]
        n141 = Unbundle(w312) -> ("String data out"=w303:string, w302:string, w301:string, w300:string)
        n142 = Unbundle(w356) -> ("String"=w305:string, "String"=w359:string, "String"=w358:string)
        n143 = Unbundle(w296) -> ("String"=w295:string, "String"=w294:string)
        n144 = Unbundle(w263) -> ("pressure"=w350:string, "RH"=w349:string, "gas flow"=w348:string, "vapor flow"=w347:string)
        n145 = Unbundle ("arduino 1-6")(w244) -> ("mean"=w248:string, "mean"=w355:string, "mean"=w354:string, "mean"=w353:string, "mean"=w352:string, "mean"=w246:string)
        n146 = Increment(x=w250) -> (x+1=w249:i32)
        n147 = Build Array(w357, w304, w303, w302, w301, w300, w305, w359, w358, w295, w294, w350, w349, w348, w347, w247, w248, w355, w354, w353, w352, w246) -> (w365:string[])
        n148 = property on="Current\nstep" class="DigNum (strict)"("Value"=w249) -> ()  [unwired: 2 in, 2 out]
        "State date/time" <- w298
        "K-2420" <- cluster{"Resistance":sgl} {"Resistance"=0.0} ("K-2420")
      }
      n149 = Unbundle(w79) -> ("Boolean"=w78:bool, "VISA out"=w77:refnum<visa-resource-name>, "error out"=w76:errorcluster)
      n150 = call-poly <vilib>:"Write To Spreadsheet File.vi"("1D data"=w48, "file path (dialog if empty)"=w64) -> ("new file path (Not A Path if cancelled)"=w68:path)  [unwired: 6 in]
      n151 = Unbundle(w57) -> (w62:bool, "VISA resource name out"=w61:refnum<visa-resource-name>, "error out"=w60:errorcluster)
      n152 = Unbundle(w27) -> ("Boolean"=w26:bool, "DAQ IDs in"=w25:T38)
      n153 = call "arduino_close_subIV.vi"("arduino 1-6 addresses and errors out"=w50, "arduinos on?"=w49) -> ()  [unwired: 10 in]
      n154 = case shown="True" w42 {
        tunnel: w41 -> [_ w91]
        tunnel: w40 -> [w88 w90]
        tunnel: [w88 w89] -> w39
        frame False {
        }
        frame True {
          n155 = call "Close.vi"("VISA resource name"=w91, "error in (no error)"=w90) -> ("error out"=w89:errorcluster)  [unwired: 17 in]
        }
      }
      n156 = flat-sequence {
        tunnel: w6 -> [w87]
        tunnel: [w87] -> w5
        frame #0 {
          n157 = property on="saving data?" class="Bool (strict)"("Value"=FALSE ("saving data?")) -> ()  [unwired: 2 in, 2 out]
        }
      }
      n158 = Unbundle(w74) -> ("Boolean"=w73:bool, "VISA resource name out"=w72:refnum<visa-resource-name>, "error out"=w71:errorcluster)
      n159 = case shown="True" w26 {
        tunnel: w25 -> [_ w118]
        tunnel: [errorcluster {"status"=FALSE, "code"=0, "source"=""} ("error out") w105] -> w34
        frame False {
        }
        frame True {
          n160 = Unbundle(w118) -> ("task out"=w117:refnum<k21>, "error out"=w116:errorcluster, "task out"=w115:refnum<k21>, "error out"=w114:errorcluster, "task out"=w113:refnum<k21>, "error out"=w112:errorcluster, "VISA Refnum out"=w111:refnum<visa-resource-name>, "error out"=w110:errorcluster)
          n161 = disable-structure shown="Disabled" {
            disable-tunnel: [w127 _] -> w109
            disable-tunnel: w117 -> [w126 _]
            disable-tunnel: w116 -> [w125 _]
            frame Disabled {
              n162 = call <vilib>:"DAQmx Stop Task.vi"("task/channels in"=w126, "error in"=w125) -> ("task out"=w128:refnum<k21>, "error out"=w129:errorcluster)  [unwired: 12 in]
              n163 = call <vilib>:"DAQmx Clear Task.vi"("task in"=w128, "error in"=w129) -> ("error out"=w127:errorcluster)  [unwired: 13 in]
            }
            frame Enabled {
            }
          }
          n164 = call <vilib>:"DAQmx Stop Task.vi"("task/channels in"=w115, "error in"=w114) -> ("task out"=w122:refnum<k21>, "error out"=w121:errorcluster)  [unwired: 12 in]
          n165 = call <vilib>:"DAQmx Stop Task.vi"("task/channels in"=w113, "error in"=w112) -> ("task out"=w123:refnum<k21>, "error out"=w124:errorcluster)  [unwired: 12 in]
          n166 = VISA Clear(VISA resource name=w111, error in (no error)=w110) -> (VISA resource name out=w120:refnum<visa-resource-name>, error out=w119:errorcluster)
          n167 = VISA Close(VISA resource name=w120, error in (no error)=w119) -> (error out=w106:errorcluster)
          n168 = call <vilib>:"DAQmx Clear Task.vi"("task in"=w122, "error in"=w121) -> ("error out"=w108:errorcluster)  [unwired: 13 in]
          n169 = call <vilib>:"DAQmx Clear Task.vi"("task in"=w123, "error in"=w124) -> ("error out"=w107:errorcluster)  [unwired: 13 in]
          n170 = Merge Errors(w109, w108, w107, w106) -> (w105:errorcluster)
        }
      }
      n171 = case shown="True" w62 {
        tunnel: w61 -> [_ w153]
        tunnel: w60 -> [w151 w152]
        tunnel: [w151 w154] -> w56
        frame False {
        }
        frame True {
          n172 = call "Enable Output.vi"("error in (no error)"=w152, "Enable Output (F:Off)"=FALSE ("Output (F:Off)"), "VISA resource name"=w153) -> ("error out"=w155:errorcluster, "VISA resource name out"=w156:refnum<visa-resource-name>)  [unwired: 7 out]
          n173 = call "Close.vi"("error in (no error)"=w155, "VISA resource name"=w156) -> ("error out"=w154:errorcluster)  [unwired: 9 out]
        }
      }
      n174 = case shown="True" w78 {
        tunnel: w76 -> [w223 w226]
        tunnel: [w223 w225] -> w80
        tunnel: w77 -> [_ w224]
        frame False {
        }
        frame True {
          n175 = call "srsQcm200Close.vi"("error in"=w226, "Visa in"=w224) -> ("error out"=w225:errorcluster)  [unwired: 3 in]
        }
      }
      n176 = call-poly <vilib>:"Write To Spreadsheet File.vi"("append to file? (new file:F)"=TRUE, "2D data"=w52, "file path (dialog if empty)"=w68) -> ()  [unwired: 5 in, 1 out]
      n177 = case shown="True" w73 {
        tunnel: w72 -> [_ w193]
        tunnel: w71 -> [w190 w192]
        tunnel: [w190 w191] -> w70
        frame False {
        }
        frame True {
          n178 = VISA Close(VISA resource name=w193, error in (no error)=w192) -> (error out=w191:errorcluster)
        }
      }
      n179 = Merge Errors(w56, w70, errorcluster {"status"=FALSE, "code"=0, "source"=""} ("error in"), w39, w80, w5) -> (w84:errorcluster)
      n180 = call <vilib>:"Simple Error Handler.vi"("error in (no error)"=w34) -> ()  [unwired: 4 in, 5 out]
      n181 = call <vilib>:"Simple Error Handler.vi"("error in (no error)"=w84) -> ()  [unwired: 4 in, 5 out]
    }
  }
  n182 = disable-structure shown="Disabled" {
    frame Disabled {
      n183 = call "Configure MeasureOhms.vi"() -> ()  [unwired: 6 in, 6 out]
    }
    frame Enabled {
    }
  }
